vi "Labview串口读写.vi"() -> ()   [LabVIEW 2018]
uses:
  <vilib>/Instr/_visa.llb/VISA Configure Serial Port (Instr).vi
panel:
  in  "串口名":refnum<visa-resource-name>="COM1"
  out "读数据":string
  in  "写数据":string
  in  "停止":bool
  in  "Write":bool
  in  "bits (8)":u16=8
  in  "波特率":u32=9600
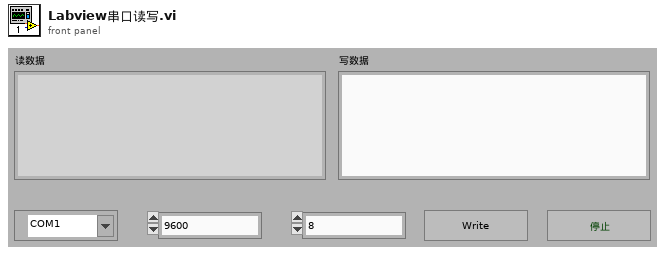
[diagram p1: front panel]
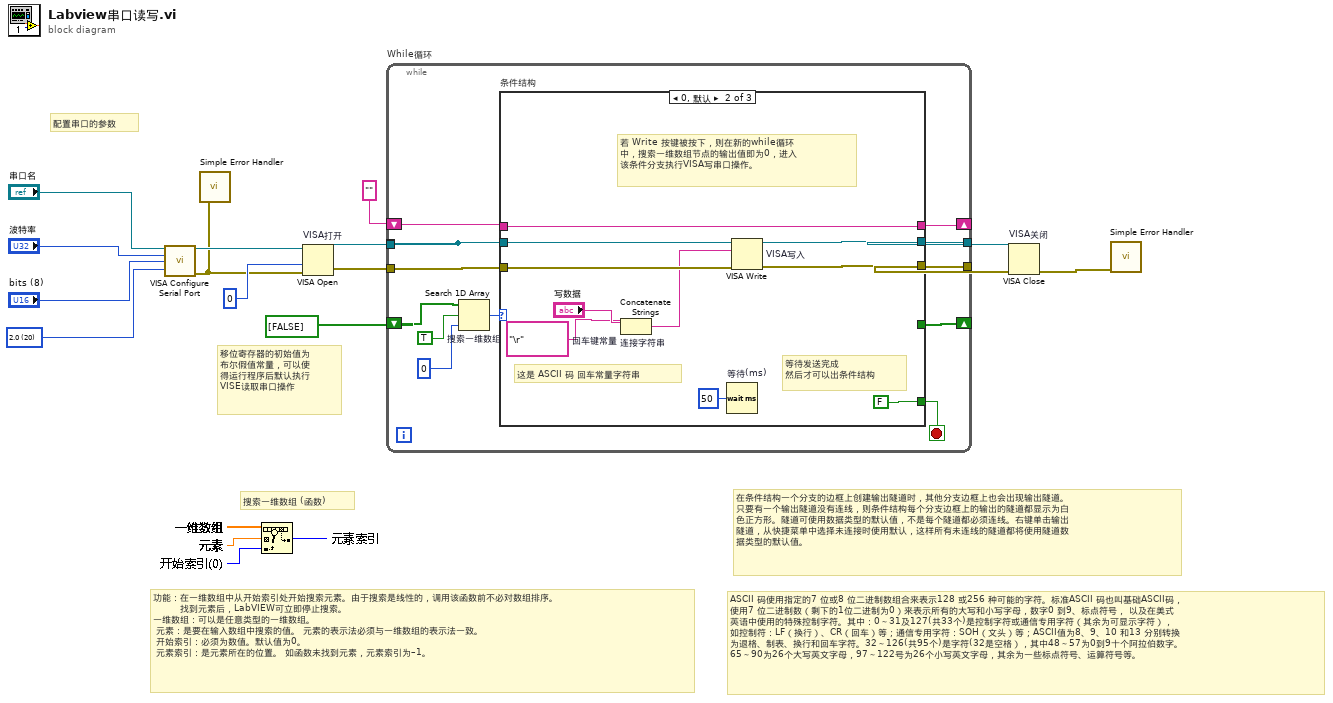
[diagram p0: block diagram]
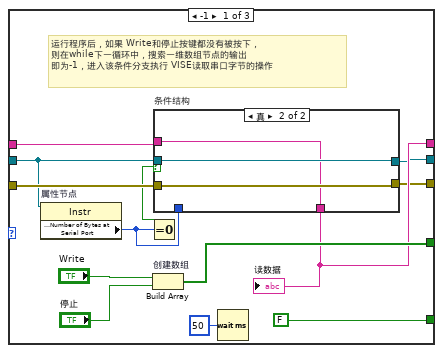
[diagram p2: hidden frame]
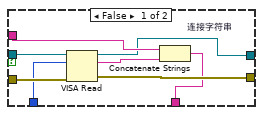
[diagram p3: hidden frame]
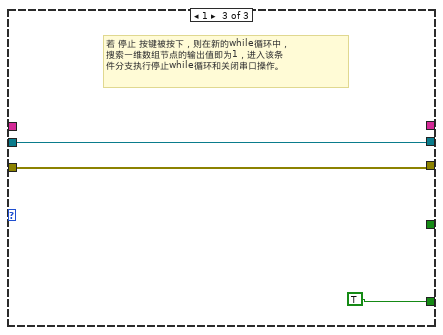
[diagram p4: hidden frame]
diagram:
  w1 = u16 20 items=["1.0"=10, "1.5"=15, "2.0"=20] ("stop bits (10: 1 bit)")
  # "配置串口的参数"
  # "ASCII 码使用指定的7 位或8 位二进制数组合来表示128 或256 种可能的字符。标准ASCII 码也叫基础ASCII码，\n使用7 位二进制数（剩下的1位二进制为0）来表示所有的大写和小写字母，数字0 到9、标点符号， 以及在美式\n英语中使用的特殊控制字符。其中：0～31及127(共33个)是控制字符或通信专用字符（其余为可显示字符），\n如控制符：LF（换行）、CR（回车）等；通信专用字符：SOH（文头）等；ASCII值为8、9、10 和13 分别转换\n为退格、制表、换行和回车字符。32～126(共95个)是字符(32是空格），其中48～57为0到9十个阿拉伯数字。\n65～90为26个大写英文字母，97～122号为26个小写英文字母，其余为一些标点符号、运算符号等。"
  # "在条件结构一个分支的边框上创建输出隧道时，其他分支边框上也会出现输出隧道。\n只要有一个输出隧道没有连线，则条件结构每个分支边框上的输出的隧道都显示为白\n色正方形。隧道可使用数据类型的默认值，不是每个隧道都必须连线。右键单击输出\n隧道，从快捷菜单中选择未连接时使用默认，这样所有未连线的隧道都将使用隧道数\n据类型的默认值。"
  # "移位寄存器的初始值为\n布尔假值常量，可以使\n得运行程序后默认执行\nVISE读取串口操作"
  # "功能：在一维数组中从开始索引处开始搜索元素。由于搜索是线性的，调用该函数前不必对数组排序。\n         找到元素后，LabVIEW可立即停止搜索。\n一维数组：可以是任意类型的一维数组。  \n 元素：是要在输入数组中搜索的值。 元素的表示法必须与一维数组的表示法一致。  \n 开始索引：必须为数值。默认值为0。  \n 元素索引：是元素所在的位置。 如函数未找到元素，元素索引为–1。"
  # "搜索一维数组 (函数)"
  n1 = call-poly "VISA Configure Serial Port"("VISA resource name"="串口名", "baud rate (9600)"="波特率", "data bits (8)"="bits (8)", "stop bits (10: 1 bit)"=w1) -> ("VISA resource name out"=w7:refnum<visa-resource-name>, "error out"=w3:errorcluster)  [unwired: 10 in]
  n2 = call <vilib>:"Simple Error Handler.vi"("error in (no error)"=w3) -> ()  [unwired: 4 in, 5 out]
  n3 = VISA Open "VISA打开"(access mode=u32 0, error in (no error)=w3, VISA resource name=w7) -> (VISA resource name=w6:refnum<visa-resource-name>, error out=w5:errorcluster)  [unwired: 2 in]
  n4 = while "While循环" {
    tunnel: [w17] -> _
    shift-right: [w15] -> _
    shift-left: bool[] [FALSE] -> [w16]
    tunnel: w5 -> [w23]
    shift-right: [w21] -> _
    shift-left: "" -> [w22]
    tunnel: [w20] -> w10
    tunnel: [w19] -> w9
    tunnel: w6 -> [w17]
    stop <- w18 stop-if-true
    n5 = Search 1D Array "搜索一维数组"(1D array=w16, element=TRUE, start index (0)=0) -> (index of element=w24:i32)
    n6 = case "条件结构" shown="0, 默认" w24 {
      tunnel: [w37 _ _] -> w15
      tunnel: w17 -> [w30 w60 w62]
      tunnel: w23 -> [w36 w59 w61]
      tunnel: w22 -> [w34 w56 _]
      tunnel: [w35 w56 _] -> w21
      tunnel: [w33 w58 w62] -> w20
      tunnel: [w32 w57 w61] -> w19
      tunnel: [FALSE FALSE TRUE] -> w18
      frame -1 {
        # "运行程序后，如果 Write和停止按键都没有被按下，\n则在while下一循环中，搜索一维数组节点的输出\n即为-1，进入该条件分支执行 VISE读取串口字节的操作"
        n7 = property on="属性节点" class="Instr"(reference=w30) -> ("Serial Settings:Number of Bytes at Serial Port"=w27:u32)  [unwired: 1 in, 2 out]
        n8 = Equal To 0?(x=w27) -> (x = 0?=w28:bool)
        n9 = Build Array "创建数组"("Write", "停止") -> (w37:bool[])
        n10 = case "条件结构" shown="真" w28 {
          tunnel: w36 -> [w47 w49]
          tunnel: [w41 w48] -> w35
          tunnel: w34 -> [w46 w48]
          tunnel: [w40 w50] -> w33
          tunnel: [w44 w49] -> w32
          tunnel: w30 -> [w43 w50]
          tunnel: w27 -> [w42 _]
          frame False {
            n11 = VISA Read ("VISA读取")(VISA resource name=w43, byte count=w42, error in (no error)=w47) -> (VISA resource name out=w40:refnum<visa-resource-name>, read buffer=w45:string, error out=w44:errorcluster)  [unwired: 1 out]
            n12 = Concatenate Strings "连接字符串"(w46, w45) -> (w41:string)
          }
          frame True {
          }
        }
        "读数据" <- w35
        n13 = Wait (ms)(milliseconds to wait=u32 50) -> ()  [unwired: 1 out]
      }
      frame 0, Default {
        w51 = "\r"  # 回车键常量
        # "等待发送完成\n然后才可以出条件结构"
        # "这是 ASCII 码 回车常量字符串"
        # "若 Write 按键被按下，则在新的while循环\n中，搜索一维数组节点的输出值即为0，进入\n该条件分支执行VISA写串口操作。"
        n14 = Concatenate Strings "连接字符串"("写数据", w51) -> (w53:string)
        n15 = Wait (ms) "等待(ms)"(milliseconds to wait=u32 50) -> ()  [unwired: 1 out]
        n16 = VISA Write "VISA写入"(VISA resource name=w60, write buffer=w53, error in (no error)=w59) -> (VISA resource name out=w58:refnum<visa-resource-name>, error out=w57:errorcluster)  [unwired: 1 out]
      }
      frame 1 {
        # "若 停止 按键被按下，则在新的while循环中，\n搜索一维数组节点的输出值即为1，进入该条\n件分支执行停止while循环和关闭串口操作。"
      }
    }
  }
  n17 = VISA Close "VISA关闭"(VISA resource name=w10, error in (no error)=w9) -> (error out=w8:errorcluster)
  n18 = call <vilib>:"Simple Error Handler.vi"("error in (no error)"=w8) -> ()  [unwired: 4 in, 5 out]
